vi "ApplyLayoutToObject.vi"(5 "scaling settings":T1={"scaling factor"={"horizontal"=1.0, "vertical"=1.0}, "scale text"=FALSE} {"scaling factor"."vertical" min=0.0; "scaling factor"."horizontal" min=0.0}, 7 "properties to ignore":variant, 8 "error in (no error)":errorcluster, 10 "GObj Refnum":refnum<vi>, 11 "Splitter Layout in":refnum<class "Splitter Layout.lvclass">) -> (0 "error out":errorcluster, 3 "Splitter Layout out":refnum<class "Splitter Layout.lvclass">)   [LabVIEW 2012, in "NI_SE_Front Panel Layout.lvlib" / "Splitter Layout.lvclass"]
doc: "Apply layout information to the GObj Refnum."
uses:
  Splitter Layout.lvclass
  Scaling Factor_Options.ctl
  XY Scaling Factor.ctl
  Object Layout/Object Layout.lvclass
  Splitter Layout.lvclass/Splitter Layout.ctl
  Properties To Ignore.vi
  NI_SE_Front Panel Layout.lvlib
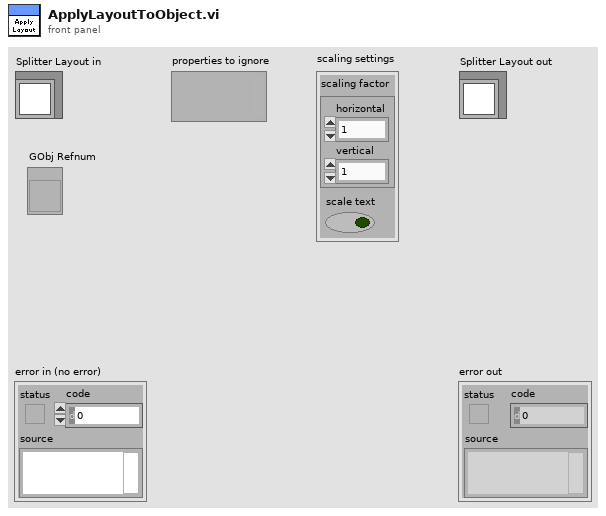
[diagram p1: front panel]
types:
  T1 = typedef "NI_SE_Front Panel Layout.lvlib/Scaling Factor_Options.ctl" = cluster{"scaling factor":T2, "scale text":bool}
  T2 = typedef "NI_SE_Front Panel Layout.lvlib/XY Scaling Factor.ctl" = cluster{"horizontal":dbl, "vertical":dbl}
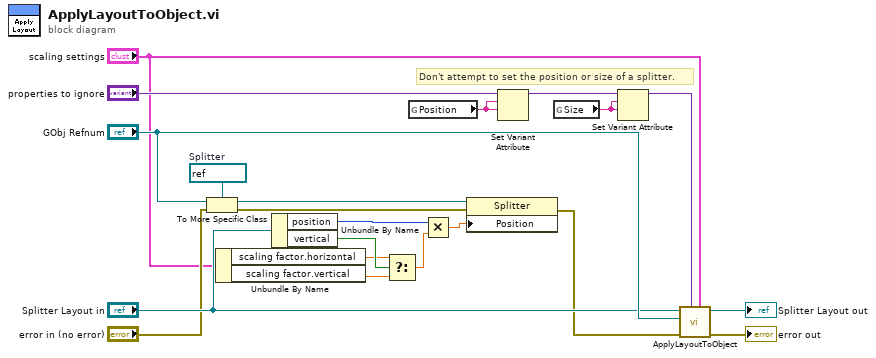
[diagram p0: block diagram]
diagram:
  w11 = refnum<vi> refnum  # Splitter
  # "Don't attempt to set the position or size of a splitter."
  n1 = To More Specific Class(target class=w11, reference="GObj Refnum", error in="error in (no error)") -> (specific class reference=w10:refnum<vi>, error out=w9:errorcluster)
  n2 = Unbundle By Name("scaling settings") -> ("scaling factor.horizontal"=w7:dbl, "scaling factor.vertical"=w6:dbl)
  n3 = Unbundle By Name("Splitter Layout in") -> ("position"=w4:i32, "vertical"=w8:bool)
  n4 = Select(t=w7, s=w8, f=w6) -> (s? t:f=w5:dbl)
  n5 = global read "Properties To Ignore.vi" "Position"() -> (w2:string)
  n6 = Multiply(x=w4, y=w5) -> (x*y=w3:dbl)
  n7 = property class="Splitter"(reference=w10, error in=w9, "Position"=w3) -> (error out=w19:errorcluster)  [unwired: 1 out]
  n8 = Set Variant Attribute(Variant="properties to ignore", name=w2, value=w2) -> (Variant out=w13:variant)  [unwired: 1 in, 2 out]
  n9 = global read "Properties To Ignore.vi" "Size"() -> (w1:string)
  n10 = Set Variant Attribute(Variant=w13, name=w1, value=w1) -> (Variant out=w12:variant)  [unwired: 1 in, 2 out]
  n11 = call-parent "ApplyLayoutToObject.vi"("scaling settings"="scaling settings", "properties to ignore"=w12, "error in (no error)"=w19, "GObj Refnum"="GObj Refnum", "Object Layout in"="Splitter Layout in") -> ("error out"=→"error out":errorcluster, "Object Layout out"=→"Splitter Layout out":refnum<class "Splitter Layout.lvclass">)  [unwired: 5 in]
